vi "Blank Module Data - Inputs (Constant).vi"() -> (0 "Blank Module Data - Inputs":T1)   [LabVIEW 2023, in "Error Manager.lvlib" / "New Error Window.lvlib"]
doc: "Outputs a \"blank\" or empty cluster. Use this to initialise, clear or reset the cluster to a known value.\n\n\"blank\" is used to mean default, empty or initial values."
uses:
  New Error Window.lvlib
  Module Data - Inputs (cluster).ctl
panel:
  # "Development\ncontrols/indicators useful for development and testing, but which are not outputs of the VI"
  # "Input\nInputs to the VI"
  # "Output\nOutputs of the VI"
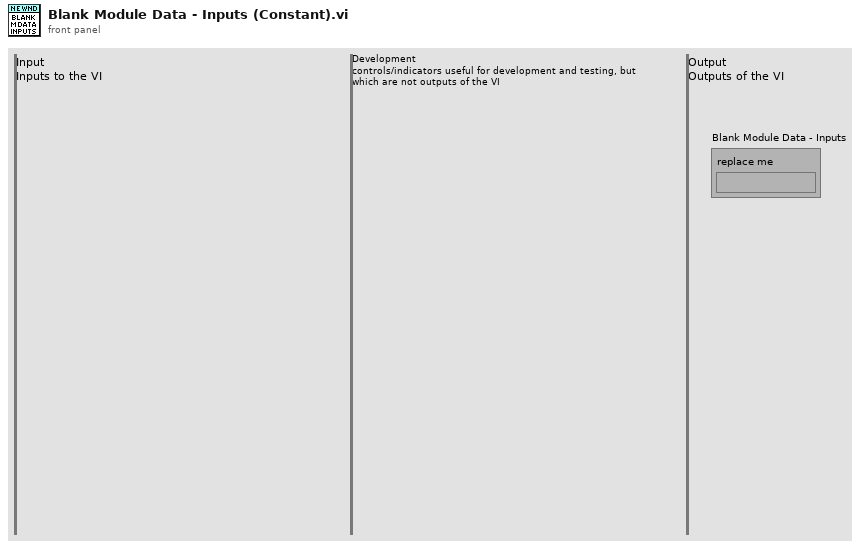
[diagram p1: front panel]
types:
  T1 = typedef "Error Manager.lvlib/New Error Window.lvlib/Module Data - Inputs (cluster).ctl" = cluster{"replace me":string}
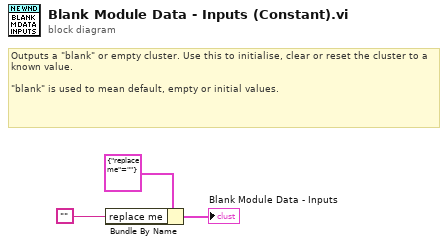
[diagram p0: block diagram]
diagram:
  # "Outputs a \"blank\" or empty cluster. Use this to initialise, clear or reset the cluster to a known value.\n\n\"blank\" is used to mean default, empty or initial values."
  n1 = Bundle By Name(cluster=T1 {"replace me"=""} ("Inputs"), "replace me"="") -> (→"Blank Module Data - Inputs":T1)
